vi "Binary to Octal.vi"(11 "Binary Numbers (0 or 1)":i64 format="%b") -> (3 "Octal Values":u32 format="%o")   [LabVIEW 2020]
doc: "This VI will convert Binary Values to Octal Values."
panel:
  out "error out":errorcluster
  in  "error in":errorcluster
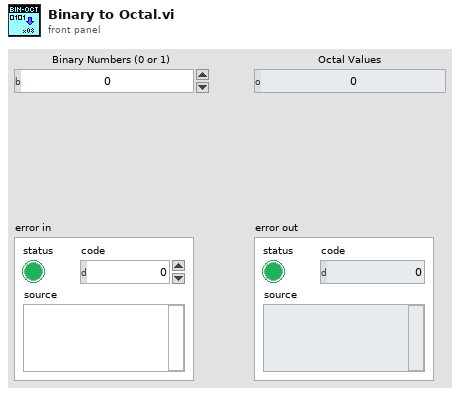
[diagram p1: front panel]
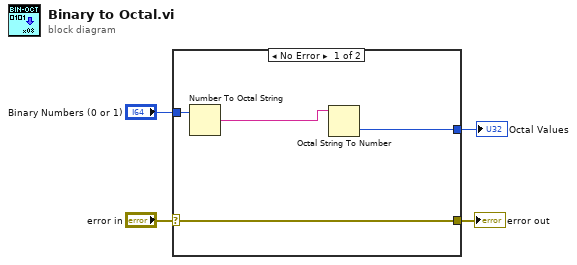
[diagram p0: block diagram]
diagram:
  n1 = case shown="No Error" "error in" {
    selector: "error in" -> [w5 w9]
    tunnel: "Binary Numbers (0 or 1)" -> [w7 _]
    tunnel: [w6 _] -> w3
    tunnel: [w5 w9] -> w1
    frame No Error {
      n2 = Number To Octal String(2:w7) -> (0:w8:string)  [unwired: 1 in]
      n3 = Octal String To Number(4:w8) -> (0:w6:u32)  [unwired: 2 in, 1 out]
    }
    frame Error {
    }
  }
  "Octal Values" <- w3
  "error out" <- w1
